vi "Periodic Tasks.vi"() -> ()   [LabVIEW 2012]
doc: "This VI runs in parallel to other tasks. It can contain as many user-defined periodic loops as you need. These can carry out PID or other sorts of timed response."
panel:
  in  "RPM Control":dbl
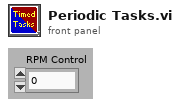
[diagram p1: front panel]
types:
  T1 = typedef "WPI_CounterDevRef.ctl" = cluster{"DevStatus":errorcluster, "CntIndex":T2}
  T2 = typedef "FPGA_CounterCtrSystemIndex.ctl" = enum8{"Ctr 0", "Ctr 1", "Ctr 2", "Ctr 3", "Ctr 4", "Ctr 5", "Ctr 6", "Ctr 7", "Invalid"}
  T3 = typedef "WPI_MotorControlDeviceRef.ctl" = cluster{"DeviceStatus":errorcluster, "Type":enum16{"PWM", "CAN"}, "PWM":cluster{"Digital Module":T4, "PWM Channel":T5, "DeadBand":T6}, "CAN":cluster{"Device Number":u8, "Control Mode":T7, "Semaphore":T8, "Max Vout":dbl}, "Invert":bool, "TransformRef":T9, "InvTransformRef":T9}
  T4 = typedef "FPGA_TypedefDigitalModule.ctl" = enum16{"Digital Module 1", "Digital Module 2"}
  T5 = typedef "FPGA_DIOPWMChannel.ctl" = enum8{"PWM 1", "PWM 2", "PWM 3", "PWM 4", "PWM 5", "PWM 6", "PWM 7", "PWM 8", "PWM 9", "PWM 10", "Invalid"}
  T6 = typedef "WPI_PWMDeadband.ctl" = cluster{"Name":string, "maxPositivePwm":i32, "minPositivePwm":i32, "centerPwm":i32, "maxNegativePwm":i32, "minNegativePwm":i32, "angularRange":u16}
  T7 = typedef "WPI_CANJaguar_ControlMode.ctl" = enum8{"Percent VBus", "Current", "Speed", "Position", "Voltage"}
  T8 = typedef "Semaphore RefNum" = refnum<k1>
  T9 = typedef "WPI_PWMTransform_ConPane.ctl" = refnum<vi>
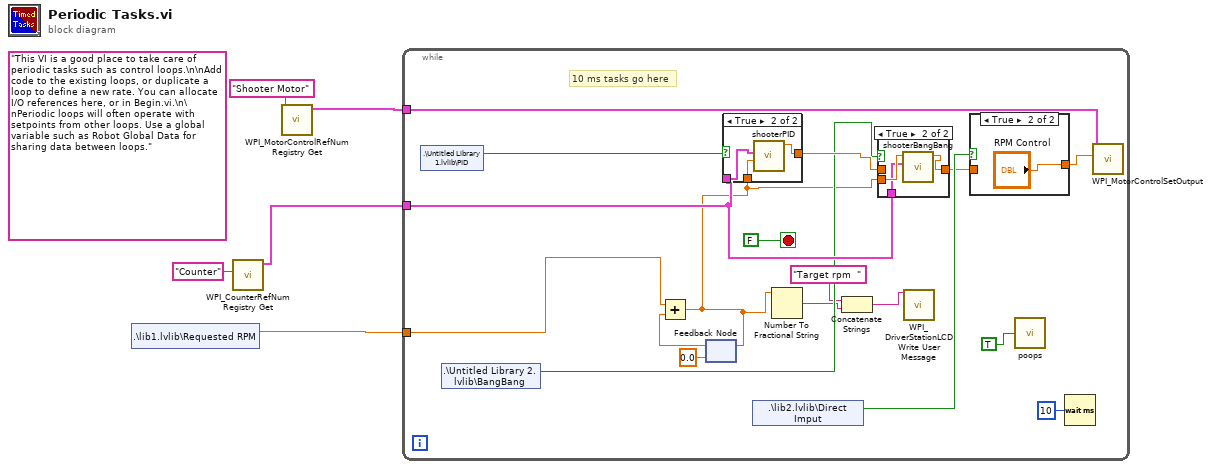
[diagram p0: block diagram]
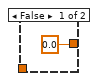
[diagram p4: hidden frame]
diagram:
  (unwired) "This VI is a good place to take care of periodic tasks such as control loops.\n\nAdd code to the existing loops, or duplicate a loop to define a new rate. You can allocate I/O references here, or in Begin.vi.\n\nPeriodic loops will often operate with setpoints from other loops. Use a global variable such as Robot Global Data for sharing data between loops."
  n1 = shared-variable ".\\lib1.lvlib\\Requested RPM"() -> (w1:dbl)  [unwired: 1 in, 1 out]
  n2 = call <vilib>:"WPI_CounterRefNum Registry Get.vi"("refnum name"="Counter") -> ("CounterDevRef"=w5:T1)  [unwired: 9 in, 1 out]
  n3 = call <vilib>:"WPI_MotorControlRefNum Registry Get.vi"("refnum name"="Shooter Motor") -> ("MotorControlDevRef"=w4:T3)  [unwired: 9 in, 1 out]
  n4 = while {
    tunnel: w5 -> [w15]
    tunnel: w4 -> [w20]
    tunnel: w1 -> [w19]
    stop <- FALSE stop-if-true
    # "10 ms tasks go here"
    n5 = shared-variable ".\\Untitled Library 1.lvlib\\PID"() -> (w21:bool)  [unwired: 1 in, 1 out]
    n6 = shared-variable ".\\Untitled Library 2.lvlib\\BangBang"() -> (w14:bool)  [unwired: 1 in, 1 out]
    n7 = feedback #1(0.0) -> (w18:dbl)
    n8 = Add(x=w19, y=w18) -> (x+y=w10:dbl)
    n9 = feedback-in #1(w10) -> ()
    n10 = case shown="True" w21 {
      tunnel: w15 -> [_ w33]
      tunnel: [0.0 w32] -> w16
      tunnel: w10 -> [_ w31]
      frame False {
      }
      frame True {
        n11 = call "shooterPID.vi"("rpmTarget"=w31, "CounterDevRef"=w33) -> ("output"=w32:dbl)  [unwired: 9 in]
      }
    }
    n12 = shared-variable ".\\lib2.lvlib\\Direct Imput"() -> (w13:bool)  [unwired: 1 in, 1 out]
    n13 = Number To Fractional String(number=w10) -> (F-format string=w9:string)  [unwired: 3 in]
    n14 = Concatenate Strings("Target rpm  " ("string"), w9) -> (w7:string)
    n15 = case shown="True" w14 {
      tunnel: w16 -> [w26 _]
      tunnel: [w26 w29] -> w12
      tunnel: w10 -> [_ w28]
      tunnel: w15 -> [_ w27]
      frame False {
      }
      frame True {
        n16 = call "shooterBangBang.vi"("CounterDevRef in"=w27, "rpmTarget"=w28) -> ("Output"=w29:dbl)  [unwired: 9 in]
      }
    }
    n17 = call <vilib>:"WPI_DriverStationLCDWrite User Message.vi"("line text"=w7) -> ()  [unwired: 14 in, 1 out]
    n18 = case shown="True" w13 {
      tunnel: w12 -> [w24 _]
      tunnel: [w24 "RPM Control"] -> w11
      frame False {
      }
      frame True {
      }
    }
    n19 = call "poops.vi"("enabled?"=TRUE) -> ()  [unwired: 2 in]
    n20 = Wait (ms)(milliseconds to wait=u32 10) -> ()  [unwired: 1 out]
    n21 = call <vilib>:"WPI_MotorControlSetOutput.vi"("Output"=w11, "MotorControlDevRef"=w20) -> ()  [unwired: 7 in, 3 out]
  }
